vi "File Column Headers.vi"() -> (3 "Column Header":string[][](array[string]))   [LabVIEW 2017]
uses:
  SubVI - Global.vi
panel:
  out "Test Info":string[](array[string])
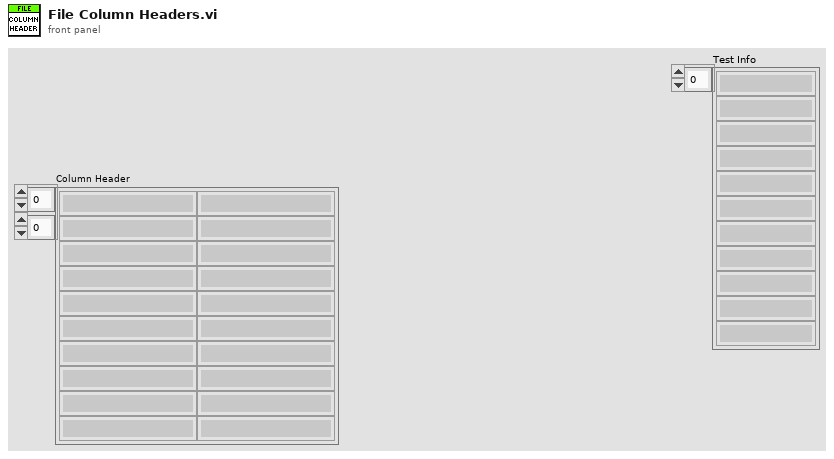
[diagram p1: front panel]
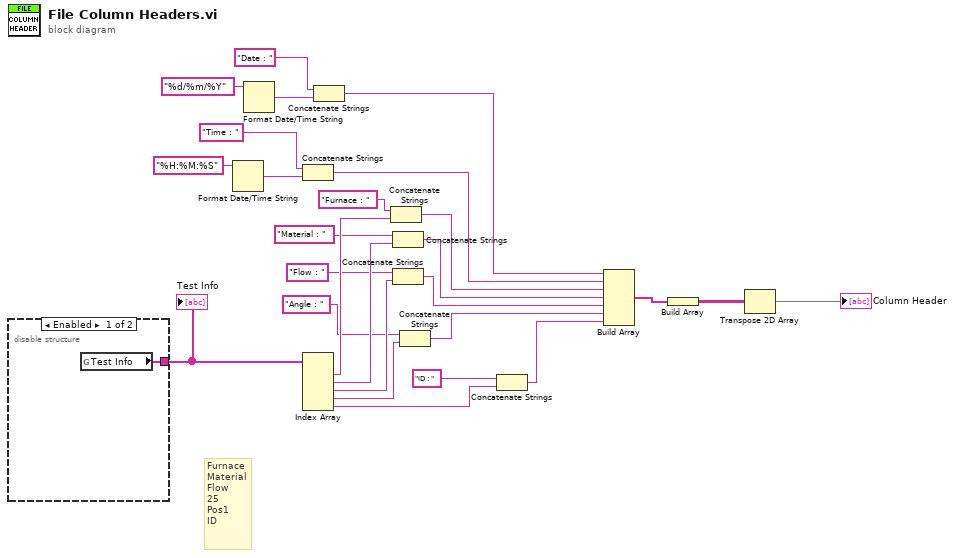
[diagram p0: block diagram]
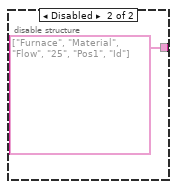
[diagram p2: hidden frame]
diagram:
  # "Furnace\nMaterial\nFlow\n25\nPos1\nID"
  n1 = disable-structure shown="Enabled" {
    disable-tunnel: [w28 string[] ["Furnace", "Material", "Flow", "25", "Pos1", "Id"] ("Test Info")] -> w20
    frame Enabled {
      n2 = global read "SubVI - Global.vi" "Test Info"() -> (w28:string[])
    }
    frame Disabled {
    }
  }
  "Test Info" <- w20
  n3 = Format Date/Time String(time format string (%c)="%H:%M:%S") -> (date/time string=w23:string)  [unwired: 2 in]
  n4 = Format Date/Time String(time format string (%c)="%d/%m/%Y") -> (date/time string=w24:string)  [unwired: 2 in]
  n5 = Concatenate Strings("Time : ", w23) -> (w18:string)
  n6 = Index Array(array=w20) -> (element #1=w14:string, element #2=w10:string, element #3=w7:string, element #4=w4:string, element #5=w2:string)  [unwired: 5 in]
  n7 = Concatenate Strings("Date : ", w24) -> (w19:string)
  n8 = Concatenate Strings("Furnace : " ("string"), w14) -> (w13:string)
  n9 = Concatenate Strings("Material : " ("string"), w10) -> (w9:string)
  n10 = Concatenate Strings("Flow : " ("string"), w7) -> (w6:string)
  n11 = Concatenate Strings("Angle : " ("string"), w4) -> (w3:string)
  n12 = Concatenate Strings("ID : " ("element"), w2) -> (w1:string)
  n13 = Build Array(w19, w18, w13, w9, w6, w3, w1) -> (w27:string[])
  n14 = Build Array(w27) -> (w16:string[][])
  n15 = Transpose 2D Array(2D array=w16) -> (transposed array=→"Column Header":string[][])
